vi "3-Bit Down Counter Controller.vi"(7 "Input":fxp<+,3,3>, 8 "Decrement?":bool, 9 "Load?":bool, 11 "Value":fxp<+,3,3>) -> (3 "Value+":fxp<+,3,3>)   [LabVIEW 2016]
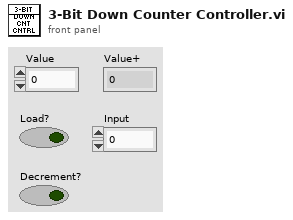
[diagram p1: front panel]
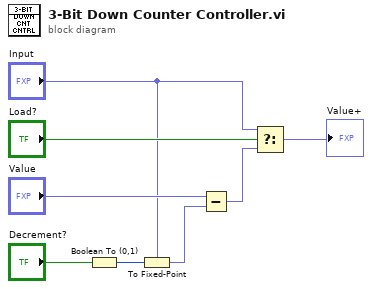
[diagram p0: block diagram]
diagram:
  n1 = Boolean To (0,1)(Boolean="Decrement?") -> (0, 1=w3:i16)
  n2 = To Fixed-Point(fixed-point type="Input", number=w3) -> (fixed-point=w2:fxp<+,3,3>)
  n3 = Subtract(x="Value", y=w2) -> (x-y=w5:fxp<+,3,3>)
  n4 = Select(t="Input", s="Load?", f=w5) -> (s? t:f=→"Value+":fxp<+,3,3>)
